vi "File List Read Files.vi"(11 "File List in":refnum<class "File List.lvclass">) -> (2 "Files":path[](array[path]), 3 "File List out":refnum<class "File List.lvclass">)   [LabVIEW 2011, in "COSYLib.lvlib" / "File List.lvclass"]
doc: "Returns all the files in the list."
uses:
  File List.lvclass
  File List.lvclass/File List.ctl
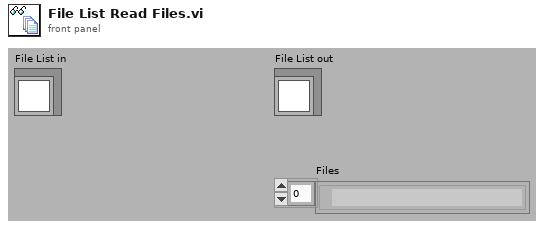
[diagram p1: front panel]
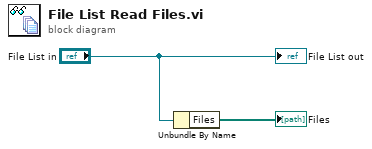
[diagram p0: block diagram]
diagram:
  n1 = Unbundle By Name("File List in") -> ("Files"=→"Files":path[])
  "File List out" <- "File List in"
